vi "Alarm interface.vi"(8 "错误输入（无错误）":errorcluster, 11 "簇":T1) -> (0 "错误输出":errorcluster)   [LabVIEW 2016, in "斯坦道CODMn.lvlib"]
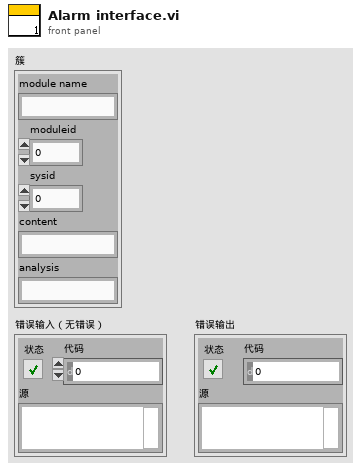
[diagram p1: front panel]
types:
  T1 = cluster{"module name":string, "moduleid":i32, "sysid":i32, "content":string, "analysis":string}
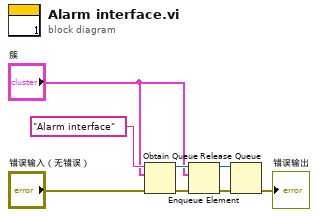
[diagram p0: block diagram]
diagram:
  n1 = Obtain Queue(name (unnamed)="Alarm interface" ("名称（未命名）"), element data type="簇", error in (no error)="错误输入（无错误）") -> (queue out=w5:refnum<queue>, error out=w6:errorcluster)  [unwired: 2 in, 1 out]
  n2 = Enqueue Element(queue=w5, element="簇", error in (no error)=w6) -> (queue out=w7:refnum<queue>, error out=w8:errorcluster)  [unwired: 1 in, 1 out]
  n3 = Release Queue(queue=w7, error in (no error)=w8) -> (error out=→"错误输出":errorcluster)  [unwired: 1 in, 2 out]
